vi "rwr_Get Shutdown Data.vi"(4 "Show in Debugger?":bool=TRUE, 6 "Message Priority":T1=enum."Normal", 7 "Caller in":refnum<class "Worker.lvclass">, 8 "error in":errorcluster, 9 "Data in":T5, 10 "timeout (ms)":i32=5000, 11 "Message Log in":refnum<class "Message Log.lvclass">) -> (0 "error out":errorcluster, 1 "Reply Data out":T2, 3 "dup Message Log out":refnum<class "Message Log.lvclass">, 5 "dup Caller out":refnum<class "Worker.lvclass">)   [LabVIEW 2017, in "Message Log.lvclass"]
doc: "This VI sends a <b>Public API Request with Reply</b> message to an MHL case of the Worker that owns this VI. This VI will wait until it receives a <b>Reply</b> message back from the Worker that owns this VI. If the wait time exceeds <b>timeout (ms)</b>, an error will be returned.\n---\nWorkers Public API Request w/Reply Case"
uses:
  Message Log.lvclass
  C:/Program Files (x86)/National Instruments/LabVIEW 2017/vi.lib/addons/_Workers/Library/Classes/Worker/Worker.lvclass
  <vilib>/addons/_Workers/Library/Classes/Worker/Worker.lvclass
  rwr_Get Shutdown.ctl
  rwr_Get Shutdown Data Reply.ctl
  Config Data.ctl
  <vilib>/Utility/miscctls.llb/LVRectTypeDef.ctl
  <vilib>/addons/_Workers/Library/Classes/Message/Priority.ctl
  <vilib>/addons/_Workers/Library/Classes/Worker/Worker.lvclass/Worker.ctl
  <vilib>/addons/_Workers/Library/Classes/Message/Message.lvclass
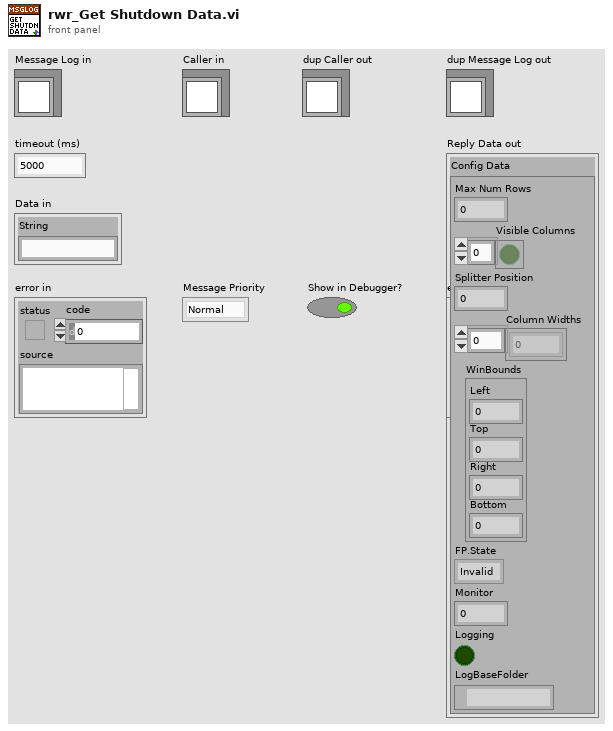
[diagram p1: front panel]
types:
  T1 = typedef "Workers.lvlib/Message.lvclass/Priority.ctl" = enum16{"Low", "Normal", "High"}
  T2 = typedef "Message Log.lvclass/rwr_Get Shutdown Data Reply.ctl" = cluster{"Config Data":T3}
  T3 = typedef "Message Log.lvclass/Config Data.ctl" = cluster{"Max Num Rows":i32, "Visible Columns":bool[], "Splitter Position":i32, "Column Widths":u32[], "WinBounds":T4, "FP.State":enum32{"Invalid", "Standard", "Closed", "Hidden", "Minimized", "Maximized"}, "Monitor":u16, "Logging":bool, "LogBaseFolder":path}
  T4 = typedef "LVRectTypeDef.ctl" = cluster{"Left":i16, "Top":i16, "Right":i16, "Bottom":i16}
  T5 = typedef "Message Log.lvclass/rwr_Get Shutdown.ctl" = cluster{"String":string}
  T6 = typedef "Workers.lvlib/Case Label.ctl" = string
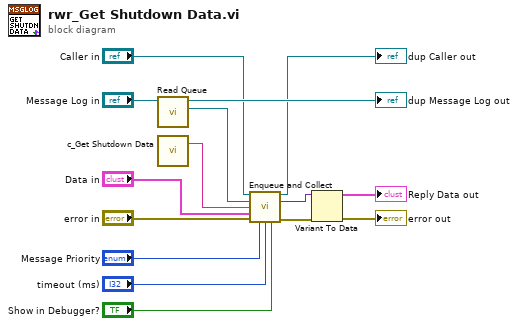
[diagram p0: block diagram]
diagram:
  n1 = call <vilib>:"Read Queue.vi"("Worker_"="Message Log in") -> ("Message Queue out"=w9:refnum<class "Message Queue.lvclass">, "dup Worker_out"=→"dup Message Log out":refnum<class "Message Log.lvclass">)  [unwired: 9 in]
  n2 = call "c_Get Shutdown Data.vi"() -> ("Case Label"=w8:T6)  [unwired: 1 in]
  n3 = call-dynamic "Enqueue and Collect.vi"("Worker"="Caller in", "Message Queue"=w9, "Case Label"=w8, "Data"="Data in", "error in (no error)"="error in", "Priority (Normal)"="Message Priority", "timeout in ms"="timeout (ms)", "Send Message to Debugger? (T)"="Show in Debugger?") -> ("dup Worker out"=→"dup Caller out":refnum<class "Worker.lvclass">, "Data out"=w4:variant, "error out"=w5:errorcluster)  [unwired: 4 in, 1 out]
  n4 = Variant To Data(error in=w5, Variant=w4) -> (data=→"Reply Data out":T2, error out=→"error out":errorcluster)  [unwired: 1 in]
